vi "DataTXTFileInfo.vi"(9 "Language":u32, 11 "file path (dialog if empty)":path caption="文件路径 （空时为对话框）") -> (0 "路径输出":path, 1 "FileInfo":string, 2 "文件类型":string)   [LabVIEW 2015]
uses:
  <vilib>/regexp/Match Regular Expression.xnode
panel:
  out "匹配子字符串":string
  out "输出 2":string
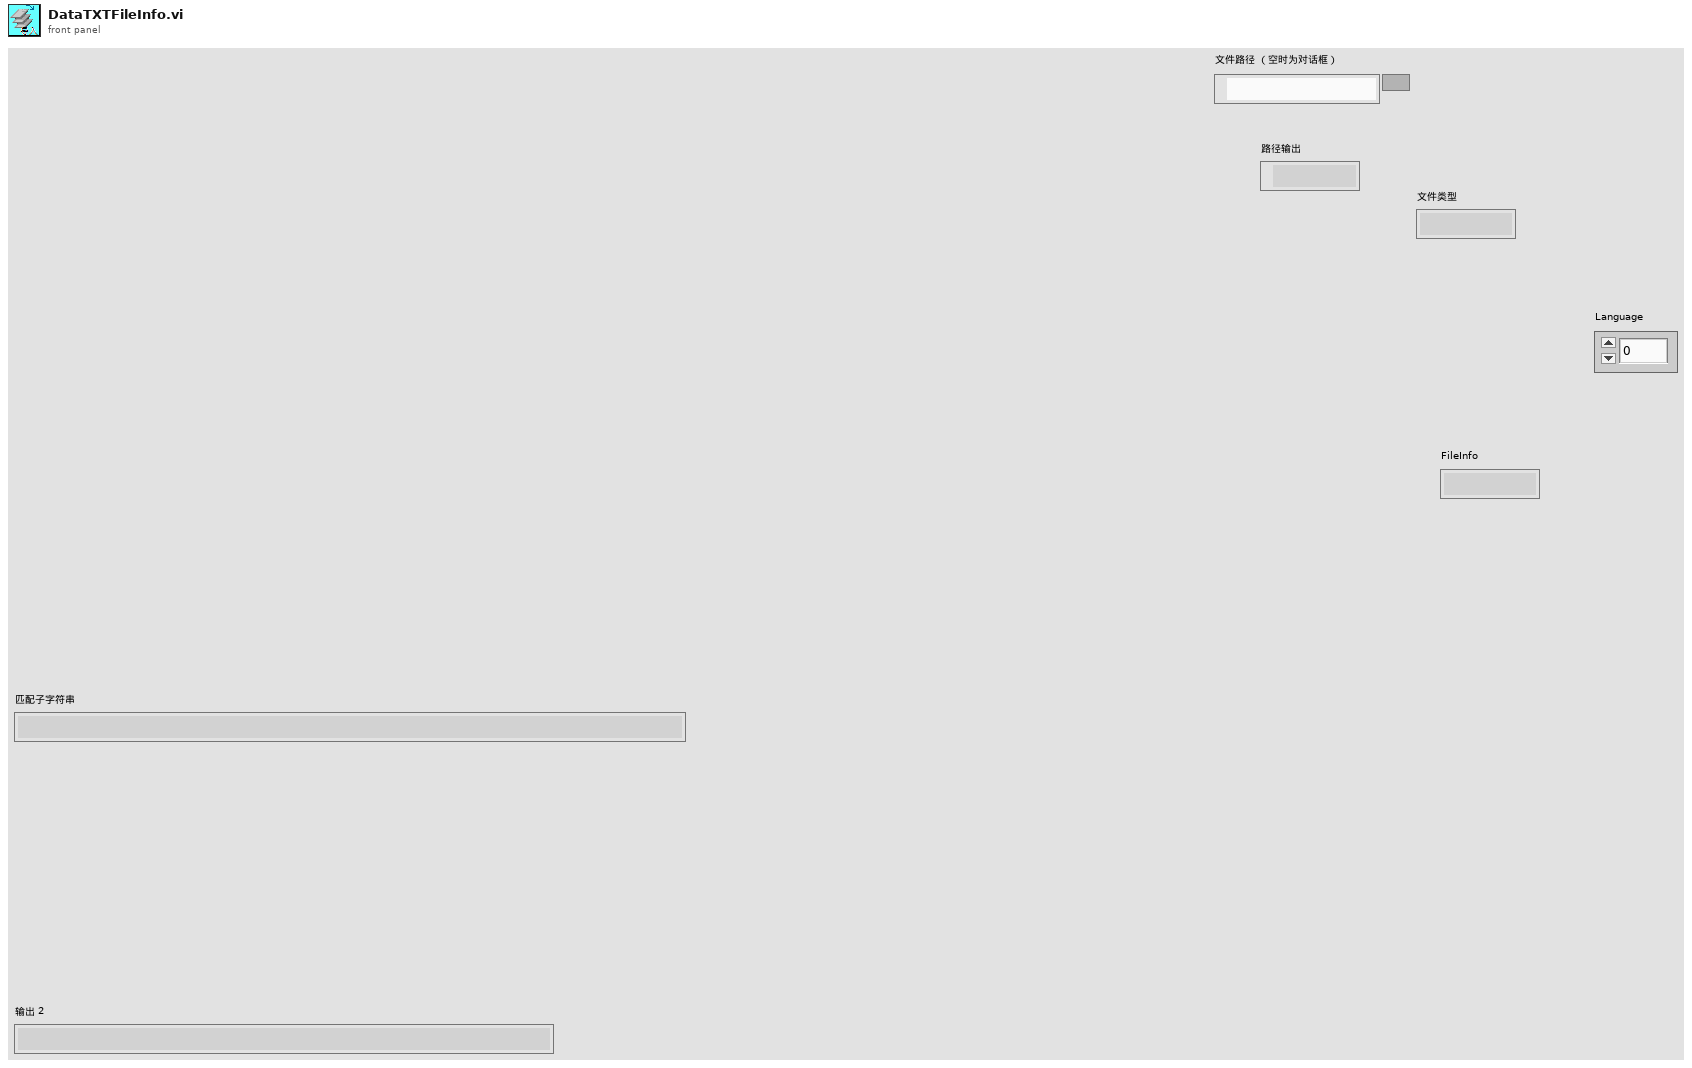
[diagram p1: front panel]
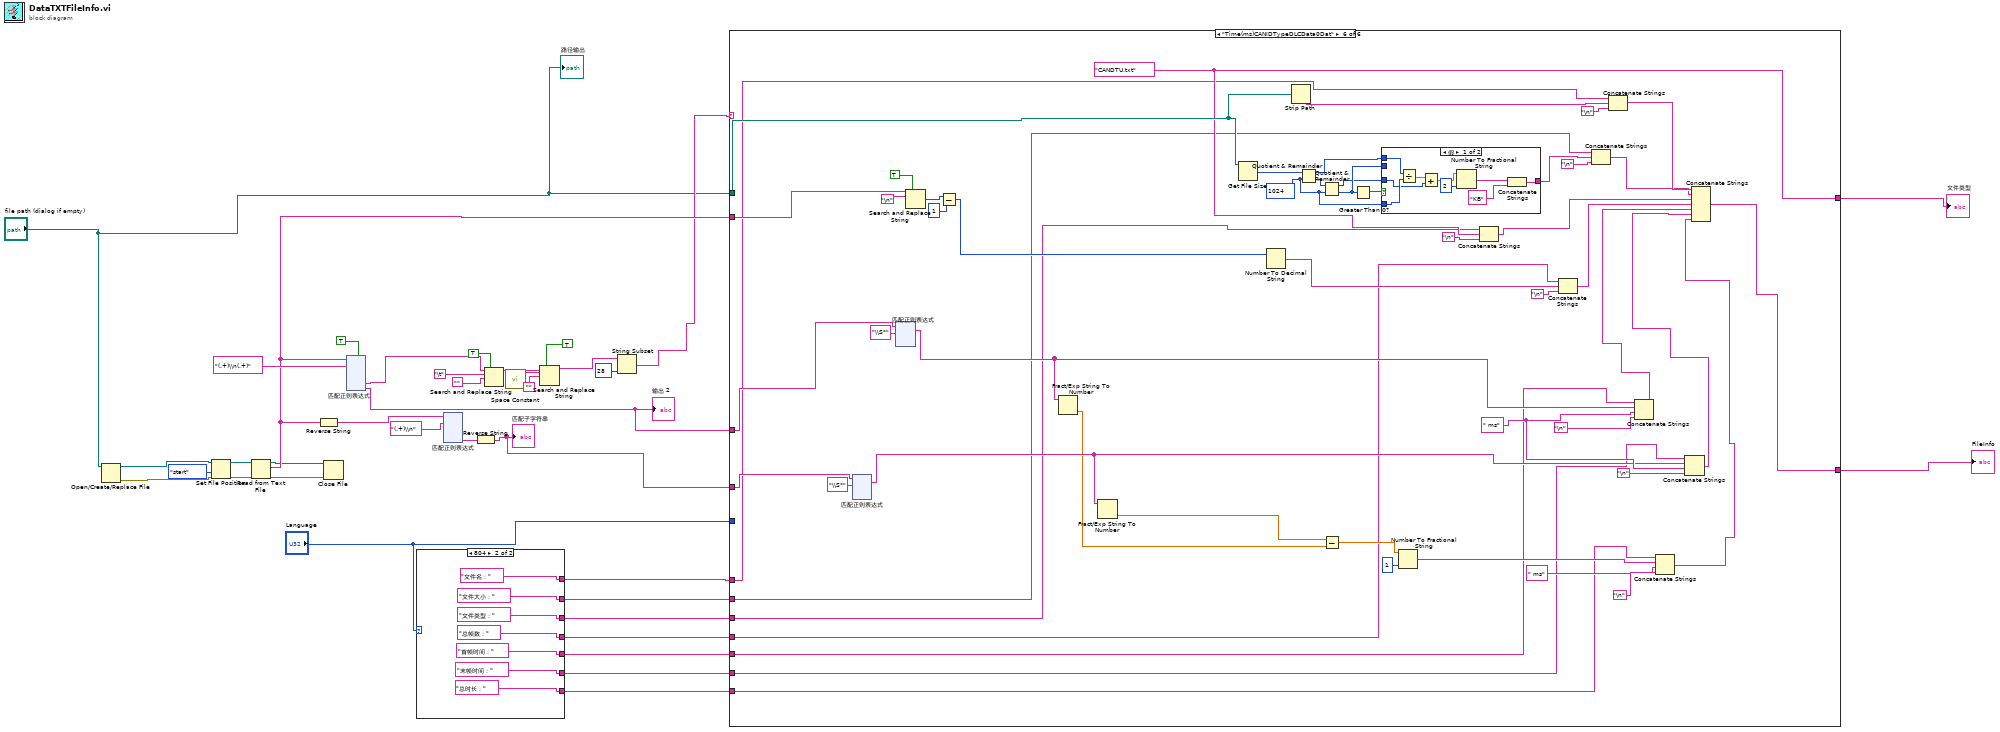
[diagram p0: block diagram]
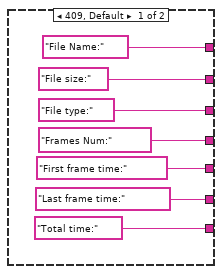
[diagram p2: hidden frame]
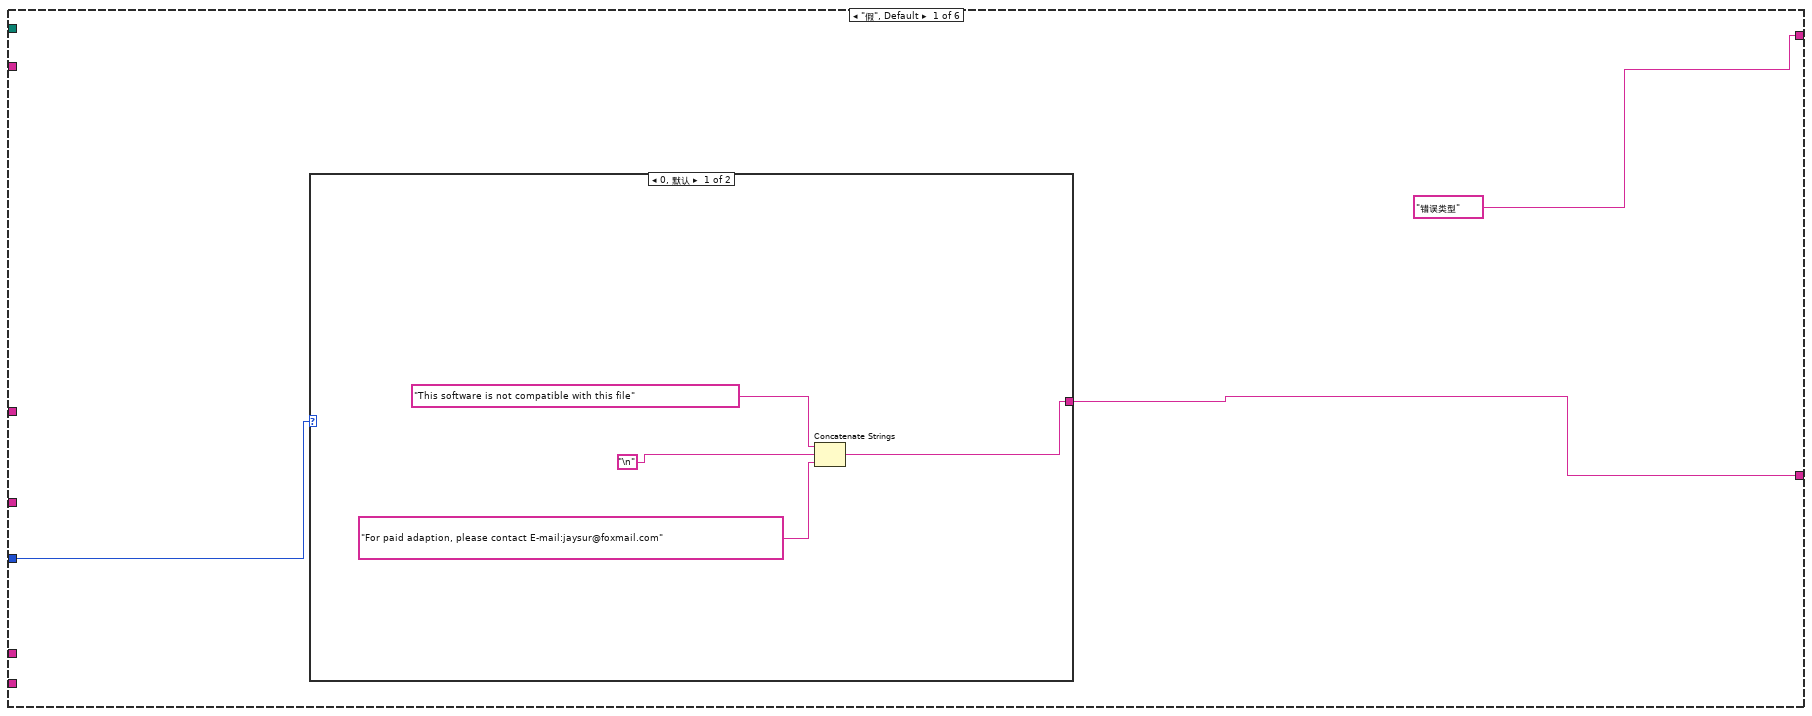
[diagram p3: hidden frame]
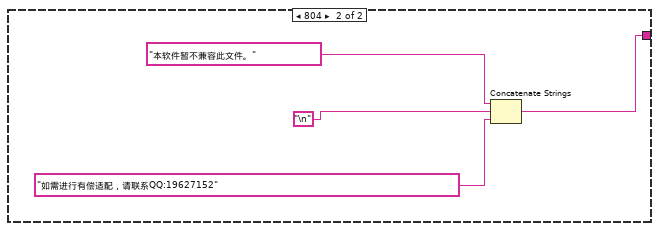
[diagram p4: hidden frame]
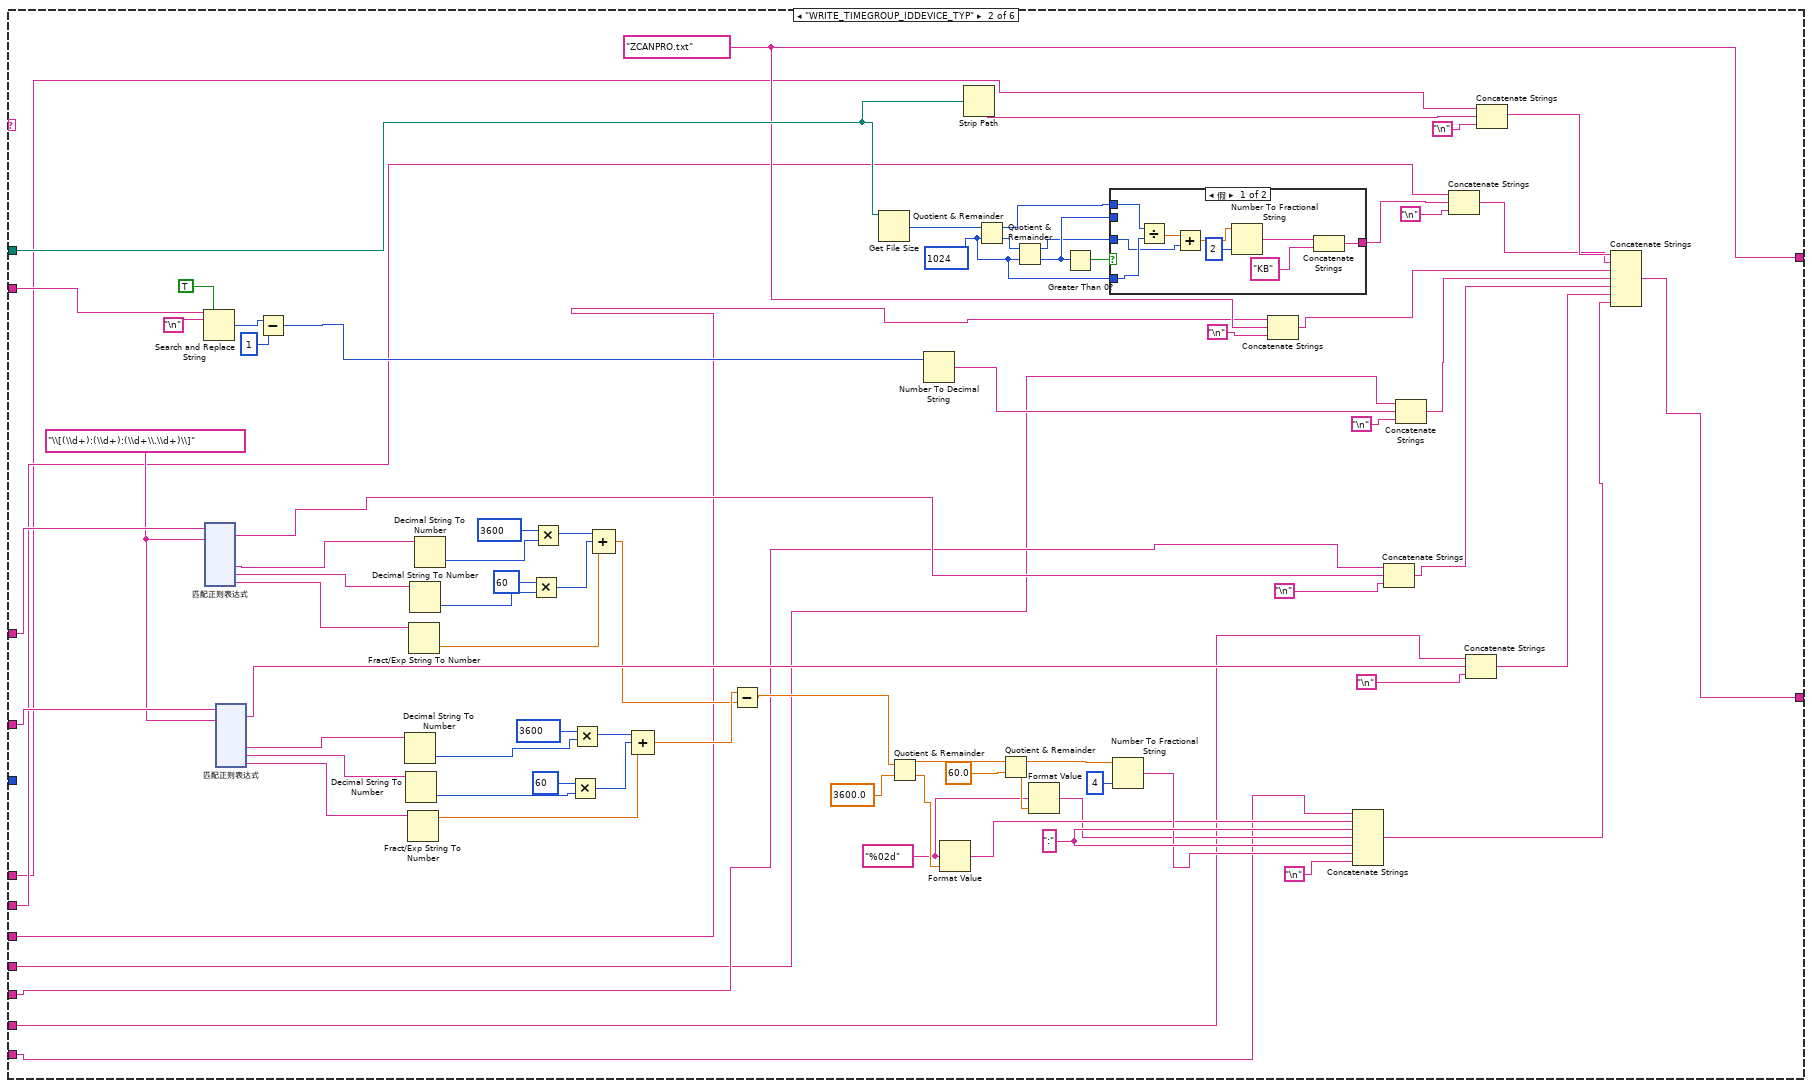
[diagram p5: hidden frame]
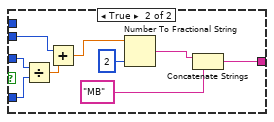
[diagram p6: hidden frame]
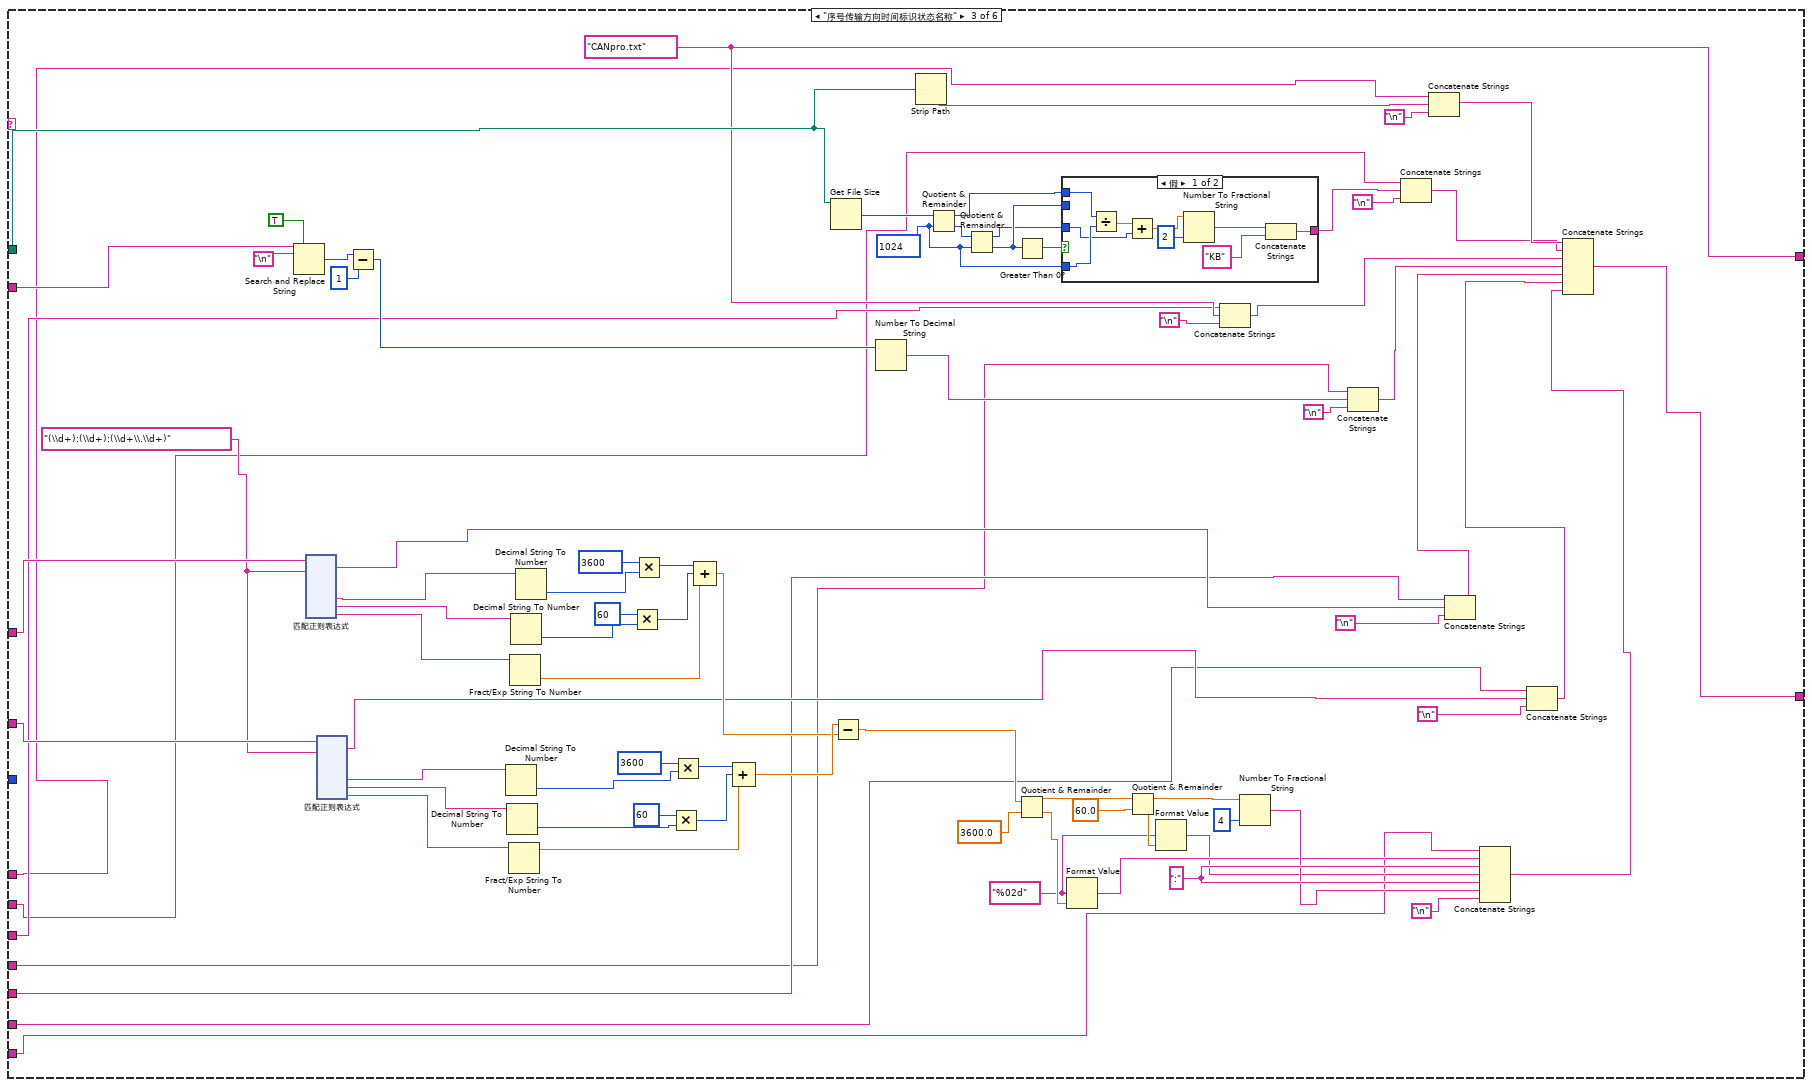
[diagram p7: hidden frame]
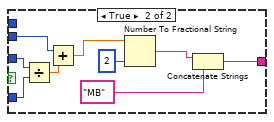
[diagram p8: hidden frame]
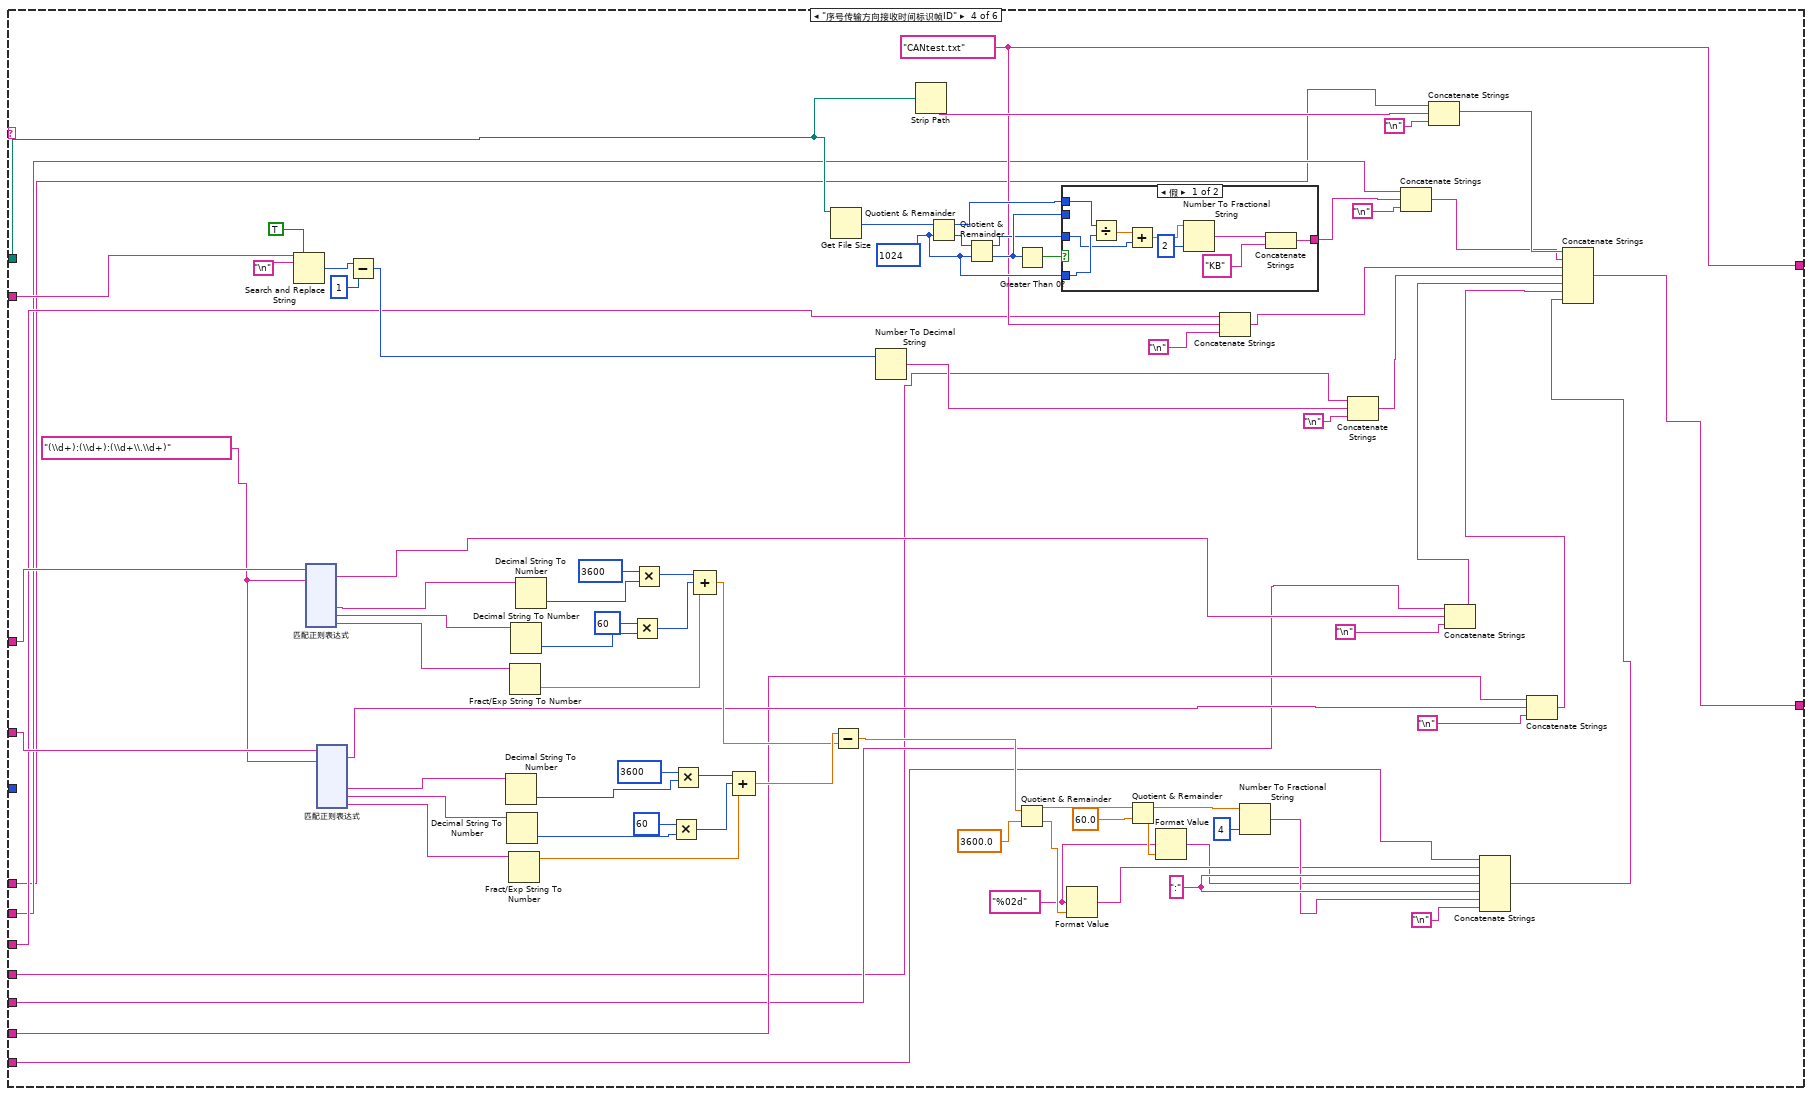
[diagram p9: hidden frame]
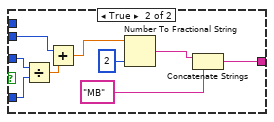
[diagram p10: hidden frame]
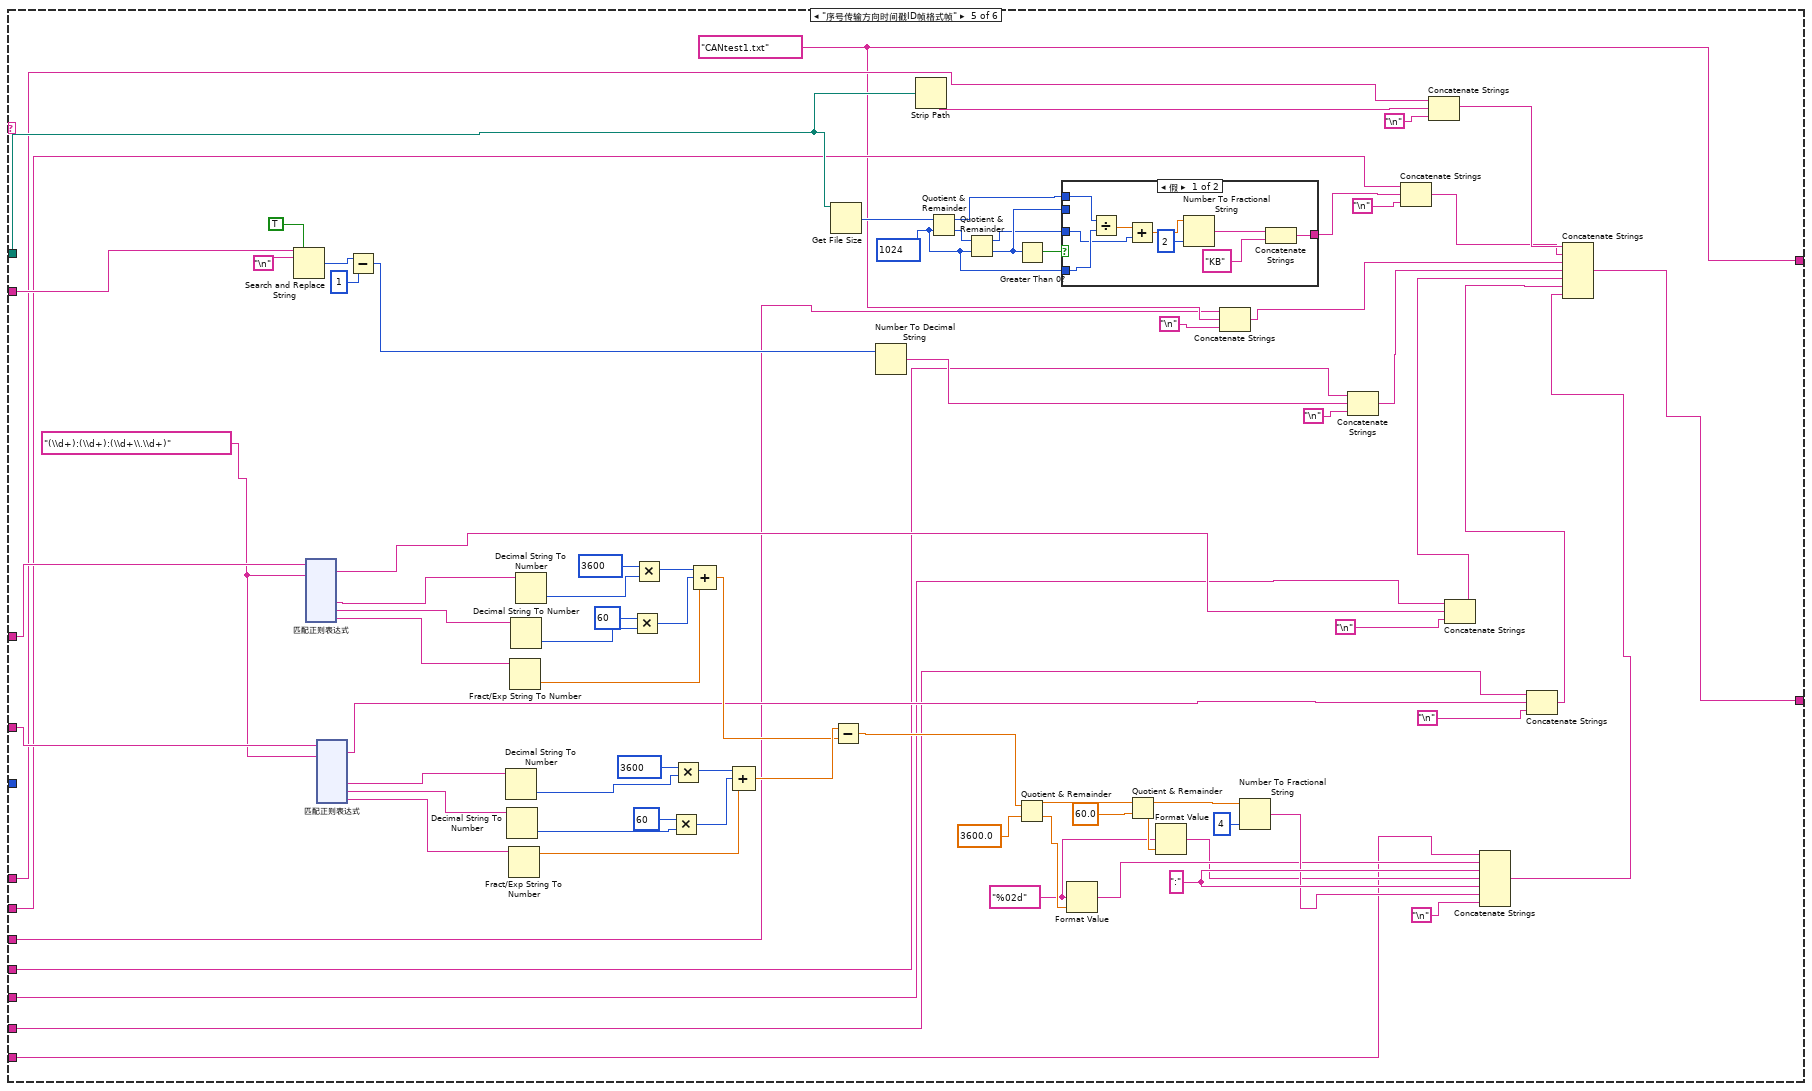
[diagram p11: hidden frame]
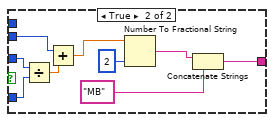
[diagram p12: hidden frame]
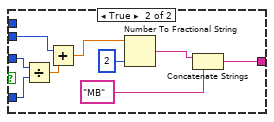
[diagram p13: hidden frame]
diagram:
  n1 = Open/Create/Replace File(file path (use dialog)="file path (dialog if empty)") -> (refnum out=w14:refnum<file>, error out=w13:errorcluster)  [unwired: 5 in, 1 out]
  n2 = Set File Position(refnum=w14, from (0:start)=enum16{"start", "end", "current"}."start" ("自（0:起始）"), error in=w13) -> (refnum out=w35:refnum<file>, error out=w33:errorcluster)  [unwired: 1 in]
  n3 = Read from Text File(file (use dialog)=w35, error in=w33) -> (refnum out=w11:refnum<file>, text=w17:string, error out=w12:errorcluster)  [unwired: 2 in, 1 out]
  n4 = Reverse String(1:w17) -> (0:w21:string)
  n5 = Close File(refnum=w11, error in=w12) -> ()  [unwired: 2 out]
  n6 = xnode "匹配正则表达式"("输入字符串"=w17, "正则表达式"="(.+)\\n(.+)", "多行？(F)"=TRUE) -> ("子匹配 1"=w28:string, "子匹配 2"=w15:string)  [unwired: 3 in, 5 out]
  "输出 2" <- w15
  n7 = case shown="804" "Language" {
    tunnel: ["Total time:" "总时长："] -> w7
    tunnel: ["Last frame time:" "末帧时间："] -> w6
    tunnel: ["First frame time:" "首帧时间："] -> w5
    tunnel: ["Frames Num:" "总帧数："] -> w4
    tunnel: ["File type:" "文件类型："] -> w3
    tunnel: ["File size:" "文件大小："] -> w2
    tunnel: ["File Name:" "文件名："] -> w1
    frame 409, Default {
    }
    frame 804 {
    }
  }
  n8 = xnode "匹配正则表达式"("输入字符串"=w21, "正则表达式"="(.+)\\n") -> ("子匹配 1"=w20:string)  [unwired: 4 in, 5 out]
  n9 = Reverse String(1:w20) -> (0:w9:string)
  "匹配子字符串" <- w9
  n10 = Search and Replace String(replace all?=TRUE ("替换全部？(F)"), input string=w28, search string="\t", replace string="") -> (result string=w26:string)  [unwired: 4 in, 3 out]
  n11 = call <vilib>:"Space Constant.vi"() -> ("String"=w25:string)
  n12 = Search and Replace String(replace all?=TRUE ("替换全部？(F)"), input string=w26, search string=w25, replace string="") -> (result string=w19:string)  [unwired: 4 in, 3 out]
  n13 = String Subset(string=w19, length (rest)=28 ("长度（剩余）")) -> (substring=w16:string)  [unwired: 1 in]
  n14 = case shown="\"Time(ms)CANIDTypeDLCData0Dat\"" w16 {
    tunnel: [w53 w109 w439 w773 w1107 w1432] -> w37
    tunnel: ["错误类型" w66 w404 w738 w1070 w1406] -> w36
    tunnel: "file path (dialog if empty)" -> [_ w105 w443 w777 w1111 w1433]
    tunnel: w17 -> [_ w100 w434 w768 w1102 w1427]
    tunnel: w15 -> [_ w96 w410 w744 w1078 w1407]
    tunnel: w9 -> [_ w98 w409 w743 w1077 w1408]
    tunnel: "Language" -> [w52 _ _ _ _ _]
    tunnel: w7 -> [_ w70 w400 w734 w1066 w1399]
    tunnel: w6 -> [_ w69 w399 w733 w1065 w1400]
    tunnel: w5 -> [_ w68 w398 w732 w1067 w1401]
    tunnel: w4 -> [_ w67 w397 w731 w1068 w1402]
    tunnel: w3 -> [_ w65 w403 w737 w1069 w1405]
    tunnel: w2 -> [_ w64 w402 w736 w1071 w1404]
    tunnel: w1 -> [_ w63 w401 w735 w1072 w1403]
    frame "假", Default {
      n15 = case shown="0, 默认" w52 {
        tunnel: [w55 w59] -> w53
        frame 0, Default {
          n16 = Concatenate Strings("This software is not compatible with this file", "\n", "For paid adaption, please contact E-mail:jaysur@foxmail.com") -> (w55:string)
        }
        frame 804 {
          n17 = Concatenate Strings("本软件暂不兼容此文件。", "\n", "如需进行有偿适配，请联系QQ:19627152") -> (w59:string)
        }
      }
    }
    frame "WRITE_TIMEGROUP_IDDEVICE_TYP" {
      w95 = "\\[(\\d+):(\\d+):(\\d+\\.\\d+)\\]"
      w114 = i64 1024 ("y")
      w131 = "%02d" ("格式字符串")
      w137 = ":"
      w66 = "ZCANPRO.txt"
      n18 = Search and Replace String(replace all?=TRUE ("替换全部？(F)"), input string=w100, search string="\n") -> (number of replacements=w102:i32)  [unwired: 5 in, 3 out]
      n19 = xnode "匹配正则表达式"("输入字符串"=w96, "正则表达式"=w95) -> ("所有匹配"=w94:string, "子匹配 1"=w93:string, "子匹配 2"=w92:string, "子匹配 3"=w91:string)  [unwired: 4 in, 4 out]
      n20 = xnode "匹配正则表达式"("输入字符串"=w98, "正则表达式"=w95) -> ("所有匹配"=w97:string, "子匹配 1"=w90:string, "子匹配 2"=w89:string, "子匹配 3"=w88:string)  [unwired: 4 in, 4 out]
      n21 = Subtract(x=w102, y=1) -> (x-y=w99:i32)
      n22 = Decimal String To Number(string=w90) -> (number=w76:i32)  [unwired: 2 in, 1 out]
      n23 = Decimal String To Number(string=w89) -> (number=w75:i32)  [unwired: 2 in, 1 out]
      n24 = Fract/Exp String To Number(string=w88) -> (number=w74:dbl)  [unwired: 3 in, 1 out]
      n25 = Fract/Exp String To Number(string=w91) -> (number=w81:dbl)  [unwired: 3 in, 1 out]
      n26 = Decimal String To Number(string=w92) -> (number=w87:i32)  [unwired: 2 in, 1 out]
      n27 = Decimal String To Number(string=w93) -> (number=w85:i32)  [unwired: 2 in, 1 out]
      n28 = Multiply(x=60, y=w87) -> (x*y=w82:i32)
      n29 = Multiply(x=3600, y=w85) -> (x*y=w83:i32)
      n30 = Multiply(x=60, y=w75) -> (x*y=w77:i32)
      n31 = Multiply(x=3600, y=w76) -> (x*y=w78:i32)
      n32 = Compound Arithmetic op=ADD(w83, w82, w81) -> (w72:dbl)
      n33 = Compound Arithmetic op=ADD(w78, w77, w74) -> (w73:dbl)
      n34 = Subtract(x=w73, y=w72) -> (x-y=w71:dbl)
      n35 = Get File Size(file=w105) -> (size (in bytes)=w117:i64)  [unwired: 1 in, 2 out]
      n36 = Quotient & Remainder(x=w71, y=3600.0) -> (x-y*floor(x/y)=w141:dbl, floor(x/y)=w134:dbl)
      n37 = Number To Decimal String(number=w99) -> (decimal integer string=w120:string)  [unwired: 1 in]
      n38 = Format Value(format string=w131, value (0)=w134) -> (output string=w135:string)  [unwired: 1 in]
      n39 = Strip Path(path=w105) -> (name=w127:string)  [unwired: 1 out]
      n40 = Quotient & Remainder(x=w117, y=w114) -> (x-y*floor(x/y)=w110:i64, floor(x/y)=w116:i64)
      n41 = Quotient & Remainder(x=w141, y=60.0) -> (x-y*floor(x/y)=w139:dbl, floor(x/y)=w133:dbl)
      n42 = Quotient & Remainder(x=w116, y=w114) -> (x-y*floor(x/y)=w112:i64, floor(x/y)=w113:i64)
      n43 = Format Value(format string=w131, value (0)=w133) -> (output string=w132:string)  [unwired: 1 in]
      n44 = Greater Than 0?(x=w113) -> (x > 0?=w115:bool)
      n45 = case shown="假" w115 {
        tunnel: w114 -> [w384 w394]
        tunnel: w113 -> [_ w392]
        tunnel: w112 -> [w382 w395]
        tunnel: [w387 w390] -> w111
        tunnel: w110 -> [w385 _]
        frame False {
          n46 = Divide(x=w385, y=w384) -> (x/y=w383:dbl)
          n47 = Add(x=w383, y=w382) -> (x+y=w381:dbl)
          n48 = Number To Fractional String(number=w381, precision (6)=i16 2 ("精度(6)")) -> (F-format string=w379:string)  [unwired: 2 in]
          n49 = Concatenate Strings(w379, "KB" ("字符串")) -> (w387:string)
        }
        frame True {
          n50 = Divide(x=w395, y=w394) -> (x/y=w393:dbl)
          n51 = Add(x=w392, y=w393) -> (x+y=w391:dbl)
          n52 = Number To Fractional String(number=w391, precision (6)=i16 2 ("精度(6)")) -> (F-format string=w389:string)  [unwired: 2 in]
          n53 = Concatenate Strings(w389, "MB") -> (w390:string)
        }
      }
      n54 = Number To Fractional String(number=w139, precision (6)=i16 4 ("精度(6)")) -> (F-format string=w136:string)  [unwired: 2 in]
      n55 = Concatenate Strings(w65, w66, "\n") -> (w124:string)
      n56 = Concatenate Strings(w70, w135, w137, w132, w137, w136, "\n") -> (w108:string)
      n57 = Concatenate Strings(w68, w94, "\n") -> (w106:string)
      n58 = Concatenate Strings(w67, w120, "\n") -> (w121:string)
      n59 = Concatenate Strings(w64, w111, "\n") -> (w118:string)
      n60 = Concatenate Strings(w69, w97, "\n") -> (w107:string)
      n61 = Concatenate Strings(w63, w127, "\n") -> (w126:string)
      n62 = Concatenate Strings(w126, w118, w124, w121, w106, w107, w108) -> (w109:string)
    }
    frame "序号传输方向时间标识状态名称" {
      w406 = "(\\d+):(\\d+):(\\d+\\.\\d+)"
      w448 = i64 1024 ("y")
      w465 = "%02d" ("格式字符串")
      w471 = ":"
      w404 = "CANpro.txt"
      n63 = Search and Replace String(replace all?=TRUE ("替换全部？(F)"), input string=w434, search string="\n") -> (number of replacements=w436:i32)  [unwired: 5 in, 3 out]
      n64 = xnode "匹配正则表达式"("输入字符串"=w410, "正则表达式"=w406) -> ("所有匹配"=w408:string, "子匹配 1"=w432:string, "子匹配 2"=w431:string, "子匹配 3"=w430:string)  [unwired: 4 in, 4 out]
      n65 = xnode "匹配正则表达式"("输入字符串"=w409, "正则表达式"=w406) -> ("所有匹配"=w407:string, "子匹配 1"=w429:string, "子匹配 2"=w428:string, "子匹配 3"=w427:string)  [unwired: 4 in, 4 out]
      n66 = Subtract(x=w436, y=1) -> (x-y=w433:i32)
      n67 = Decimal String To Number(string=w429) -> (number=w415:i32)  [unwired: 2 in, 1 out]
      n68 = Decimal String To Number(string=w428) -> (number=w414:i32)  [unwired: 2 in, 1 out]
      n69 = Fract/Exp String To Number(string=w427) -> (number=w413:dbl)  [unwired: 3 in, 1 out]
      n70 = Fract/Exp String To Number(string=w430) -> (number=w420:dbl)  [unwired: 3 in, 1 out]
      n71 = Decimal String To Number(string=w431) -> (number=w426:i32)  [unwired: 2 in, 1 out]
      n72 = Decimal String To Number(string=w432) -> (number=w424:i32)  [unwired: 2 in, 1 out]
      n73 = Multiply(x=60, y=w426) -> (x*y=w421:i32)
      n74 = Multiply(x=3600, y=w424) -> (x*y=w422:i32)
      n75 = Multiply(x=60, y=w414) -> (x*y=w416:i32)
      n76 = Multiply(x=3600, y=w415) -> (x*y=w417:i32)
      n77 = Compound Arithmetic op=ADD(w422, w421, w420) -> (w411:dbl)
      n78 = Compound Arithmetic op=ADD(w417, w416, w413) -> (w412:dbl)
      n79 = Get File Size(file=w443) -> (size (in bytes)=w451:i64)  [unwired: 1 in, 2 out]
      n80 = Subtract(x=w412, y=w411) -> (x-y=w405:dbl)
      n81 = Number To Decimal String(number=w433) -> (decimal integer string=w454:string)  [unwired: 1 in]
      n82 = Strip Path(path=w443) -> (name=w461:string)  [unwired: 1 out]
      n83 = Quotient & Remainder(x=w451, y=w448) -> (x-y*floor(x/y)=w444:i64, floor(x/y)=w450:i64)
      n84 = Quotient & Remainder(x=w450, y=w448) -> (x-y*floor(x/y)=w446:i64, floor(x/y)=w447:i64)
      n85 = Greater Than 0?(x=w447) -> (x > 0?=w449:bool)
      n86 = Quotient & Remainder(x=w405, y=3600.0) -> (x-y*floor(x/y)=w475:dbl, floor(x/y)=w468:dbl)
      n87 = case shown="假" w449 {
        tunnel: w448 -> [w718 w728]
        tunnel: w447 -> [_ w726]
        tunnel: w446 -> [w716 w729]
        tunnel: [w721 w724] -> w445
        tunnel: w444 -> [w719 _]
        frame False {
          n88 = Divide(x=w719, y=w718) -> (x/y=w717:dbl)
          n89 = Add(x=w717, y=w716) -> (x+y=w715:dbl)
          n90 = Number To Fractional String(number=w715, precision (6)=i16 2 ("精度(6)")) -> (F-format string=w713:string)  [unwired: 2 in]
          n91 = Concatenate Strings(w713, "KB" ("字符串")) -> (w721:string)
        }
        frame True {
          n92 = Divide(x=w729, y=w728) -> (x/y=w727:dbl)
          n93 = Add(x=w726, y=w727) -> (x+y=w725:dbl)
          n94 = Number To Fractional String(number=w725, precision (6)=i16 2 ("精度(6)")) -> (F-format string=w723:string)  [unwired: 2 in]
          n95 = Concatenate Strings(w723, "MB") -> (w724:string)
        }
      }
      n96 = Format Value(format string=w465, value (0)=w468) -> (output string=w469:string)  [unwired: 1 in]
      n97 = Quotient & Remainder(x=w475, y=60.0) -> (x-y*floor(x/y)=w473:dbl, floor(x/y)=w467:dbl)
      n98 = Format Value(format string=w465, value (0)=w467) -> (output string=w466:string)  [unwired: 1 in]
      n99 = Concatenate Strings(w403, w404, "\n") -> (w458:string)
      n100 = Number To Fractional String(number=w473, precision (6)=i16 4 ("精度(6)")) -> (F-format string=w470:string)  [unwired: 2 in]
      n101 = Concatenate Strings(w397, w454, "\n") -> (w455:string)
      n102 = Concatenate Strings(w402, w445, "\n") -> (w452:string)
      n103 = Concatenate Strings(w401, w461, "\n") -> (w460:string)
      n104 = Concatenate Strings(w398, w408, "\n") -> (w442:string)
      n105 = Concatenate Strings(w400, w469, w471, w466, w471, w470, "\n") -> (w440:string)
      n106 = Concatenate Strings(w399, w407, "\n") -> (w441:string)
      n107 = Concatenate Strings(w460, w452, w458, w455, w442, w441, w440) -> (w439:string)
    }
    frame "序号传输方向接收时间标识帧ID" {
      w740 = "(\\d+):(\\d+):(\\d+\\.\\d+)"
      w782 = i64 1024 ("y")
      w799 = "%02d" ("格式字符串")
      w805 = ":"
      w738 = "CANtest.txt"
      n108 = Search and Replace String(replace all?=TRUE ("替换全部？(F)"), input string=w768, search string="\n") -> (number of replacements=w770:i32)  [unwired: 5 in, 3 out]
      n109 = xnode "匹配正则表达式"("输入字符串"=w744, "正则表达式"=w740) -> ("所有匹配"=w742:string, "子匹配 1"=w766:string, "子匹配 2"=w765:string, "子匹配 3"=w764:string)  [unwired: 4 in, 4 out]
      n110 = xnode "匹配正则表达式"("输入字符串"=w743, "正则表达式"=w740) -> ("所有匹配"=w741:string, "子匹配 1"=w763:string, "子匹配 2"=w762:string, "子匹配 3"=w761:string)  [unwired: 4 in, 4 out]
      n111 = Subtract(x=w770, y=1) -> (x-y=w767:i32)
      n112 = Decimal String To Number(string=w763) -> (number=w749:i32)  [unwired: 2 in, 1 out]
      n113 = Decimal String To Number(string=w762) -> (number=w748:i32)  [unwired: 2 in, 1 out]
      n114 = Fract/Exp String To Number(string=w761) -> (number=w747:dbl)  [unwired: 3 in, 1 out]
      n115 = Fract/Exp String To Number(string=w764) -> (number=w754:dbl)  [unwired: 3 in, 1 out]
      n116 = Decimal String To Number(string=w765) -> (number=w760:i32)  [unwired: 2 in, 1 out]
      n117 = Decimal String To Number(string=w766) -> (number=w758:i32)  [unwired: 2 in, 1 out]
      n118 = Multiply(x=60, y=w760) -> (x*y=w755:i32)
      n119 = Multiply(x=3600, y=w758) -> (x*y=w756:i32)
      n120 = Multiply(x=60, y=w748) -> (x*y=w750:i32)
      n121 = Multiply(x=3600, y=w749) -> (x*y=w751:i32)
      n122 = Compound Arithmetic op=ADD(w756, w755, w754) -> (w745:dbl)
      n123 = Compound Arithmetic op=ADD(w751, w750, w747) -> (w746:dbl)
      n124 = Get File Size(file=w777) -> (size (in bytes)=w785:i64)  [unwired: 1 in, 2 out]
      n125 = Subtract(x=w746, y=w745) -> (x-y=w739:dbl)
      n126 = Number To Decimal String(number=w767) -> (decimal integer string=w788:string)  [unwired: 1 in]
      n127 = Strip Path(path=w777) -> (name=w795:string)  [unwired: 1 out]
      n128 = Quotient & Remainder(x=w785, y=w782) -> (x-y*floor(x/y)=w778:i64, floor(x/y)=w784:i64)
      n129 = Quotient & Remainder(x=w784, y=w782) -> (x-y*floor(x/y)=w780:i64, floor(x/y)=w781:i64)
      n130 = Greater Than 0?(x=w781) -> (x > 0?=w783:bool)
      n131 = Quotient & Remainder(x=w739, y=3600.0) -> (x-y*floor(x/y)=w809:dbl, floor(x/y)=w802:dbl)
      n132 = case shown="假" w783 {
        tunnel: w782 -> [w1052 w1062]
        tunnel: w781 -> [_ w1060]
        tunnel: w780 -> [w1050 w1063]
        tunnel: [w1055 w1058] -> w779
        tunnel: w778 -> [w1053 _]
        frame False {
          n133 = Divide(x=w1053, y=w1052) -> (x/y=w1051:dbl)
          n134 = Add(x=w1051, y=w1050) -> (x+y=w1049:dbl)
          n135 = Number To Fractional String(number=w1049, precision (6)=i16 2 ("精度(6)")) -> (F-format string=w1047:string)  [unwired: 2 in]
          n136 = Concatenate Strings(w1047, "KB" ("字符串")) -> (w1055:string)
        }
        frame True {
          n137 = Divide(x=w1063, y=w1062) -> (x/y=w1061:dbl)
          n138 = Add(x=w1060, y=w1061) -> (x+y=w1059:dbl)
          n139 = Number To Fractional String(number=w1059, precision (6)=i16 2 ("精度(6)")) -> (F-format string=w1057:string)  [unwired: 2 in]
          n140 = Concatenate Strings(w1057, "MB") -> (w1058:string)
        }
      }
      n141 = Format Value(format string=w799, value (0)=w802) -> (output string=w803:string)  [unwired: 1 in]
      n142 = Quotient & Remainder(x=w809, y=60.0) -> (x-y*floor(x/y)=w807:dbl, floor(x/y)=w801:dbl)
      n143 = Format Value(format string=w799, value (0)=w801) -> (output string=w800:string)  [unwired: 1 in]
      n144 = Concatenate Strings(w737, w738, "\n") -> (w792:string)
      n145 = Number To Fractional String(number=w807, precision (6)=i16 4 ("精度(6)")) -> (F-format string=w804:string)  [unwired: 2 in]
      n146 = Concatenate Strings(w731, w788, "\n") -> (w789:string)
      n147 = Concatenate Strings(w736, w779, "\n") -> (w786:string)
      n148 = Concatenate Strings(w735, w795, "\n") -> (w794:string)
      n149 = Concatenate Strings(w732, w742, "\n") -> (w776:string)
      n150 = Concatenate Strings(w734, w803, w805, w800, w805, w804, "\n") -> (w774:string)
      n151 = Concatenate Strings(w733, w741, "\n") -> (w775:string)
      n152 = Concatenate Strings(w794, w786, w792, w789, w776, w775, w774) -> (w773:string)
    }
    frame "序号传输方向时间戳ID帧格式帧" {
      w1074 = "(\\d+):(\\d+):(\\d+\\.\\d+)"
      w1116 = i64 1024 ("y")
      w1133 = "%02d" ("格式字符串")
      w1139 = ":"
      w1070 = "CANtest1.txt"
      n153 = Search and Replace String(replace all?=TRUE ("替换全部？(F)"), input string=w1102, search string="\n") -> (number of replacements=w1104:i32)  [unwired: 5 in, 3 out]
      n154 = xnode "匹配正则表达式"("输入字符串"=w1078, "正则表达式"=w1074) -> ("所有匹配"=w1076:string, "子匹配 1"=w1100:string, "子匹配 2"=w1099:string, "子匹配 3"=w1098:string)  [unwired: 4 in, 4 out]
      n155 = xnode "匹配正则表达式"("输入字符串"=w1077, "正则表达式"=w1074) -> ("所有匹配"=w1075:string, "子匹配 1"=w1097:string, "子匹配 2"=w1096:string, "子匹配 3"=w1095:string)  [unwired: 4 in, 4 out]
      n156 = Subtract(x=w1104, y=1) -> (x-y=w1101:i32)
      n157 = Decimal String To Number(string=w1097) -> (number=w1083:i32)  [unwired: 2 in, 1 out]
      n158 = Decimal String To Number(string=w1096) -> (number=w1082:i32)  [unwired: 2 in, 1 out]
      n159 = Fract/Exp String To Number(string=w1095) -> (number=w1081:dbl)  [unwired: 3 in, 1 out]
      n160 = Fract/Exp String To Number(string=w1098) -> (number=w1088:dbl)  [unwired: 3 in, 1 out]
      n161 = Decimal String To Number(string=w1099) -> (number=w1094:i32)  [unwired: 2 in, 1 out]
      n162 = Decimal String To Number(string=w1100) -> (number=w1092:i32)  [unwired: 2 in, 1 out]
      n163 = Multiply(x=60, y=w1094) -> (x*y=w1089:i32)
      n164 = Multiply(x=3600, y=w1092) -> (x*y=w1090:i32)
      n165 = Multiply(x=60, y=w1082) -> (x*y=w1084:i32)
      n166 = Multiply(x=3600, y=w1083) -> (x*y=w1085:i32)
      n167 = Compound Arithmetic op=ADD(w1090, w1089, w1088) -> (w1079:dbl)
      n168 = Compound Arithmetic op=ADD(w1085, w1084, w1081) -> (w1080:dbl)
      n169 = Get File Size(file=w1111) -> (size (in bytes)=w1119:i64)  [unwired: 1 in, 2 out]
      n170 = Subtract(x=w1080, y=w1079) -> (x-y=w1073:dbl)
      n171 = Number To Decimal String(number=w1101) -> (decimal integer string=w1122:string)  [unwired: 1 in]
      n172 = Strip Path(path=w1111) -> (name=w1129:string)  [unwired: 1 out]
      n173 = Quotient & Remainder(x=w1119, y=w1116) -> (x-y*floor(x/y)=w1112:i64, floor(x/y)=w1118:i64)
      n174 = Quotient & Remainder(x=w1118, y=w1116) -> (x-y*floor(x/y)=w1114:i64, floor(x/y)=w1115:i64)
      n175 = Greater Than 0?(x=w1115) -> (x > 0?=w1117:bool)
      n176 = Quotient & Remainder(x=w1073, y=3600.0) -> (x-y*floor(x/y)=w1143:dbl, floor(x/y)=w1136:dbl)
      n177 = case shown="假" w1117 {
        tunnel: w1116 -> [w1386 w1396]
        tunnel: w1115 -> [_ w1394]
        tunnel: w1114 -> [w1384 w1397]
        tunnel: [w1389 w1392] -> w1113
        tunnel: w1112 -> [w1387 _]
        frame False {
          n178 = Divide(x=w1387, y=w1386) -> (x/y=w1385:dbl)
          n179 = Add(x=w1385, y=w1384) -> (x+y=w1383:dbl)
          n180 = Number To Fractional String(number=w1383, precision (6)=i16 2 ("精度(6)")) -> (F-format string=w1381:string)  [unwired: 2 in]
          n181 = Concatenate Strings(w1381, "KB" ("字符串")) -> (w1389:string)
        }
        frame True {
          n182 = Divide(x=w1397, y=w1396) -> (x/y=w1395:dbl)
          n183 = Add(x=w1394, y=w1395) -> (x+y=w1393:dbl)
          n184 = Number To Fractional String(number=w1393, precision (6)=i16 2 ("精度(6)")) -> (F-format string=w1391:string)  [unwired: 2 in]
          n185 = Concatenate Strings(w1391, "MB") -> (w1392:string)
        }
      }
      n186 = Format Value(format string=w1133, value (0)=w1136) -> (output string=w1137:string)  [unwired: 1 in]
      n187 = Quotient & Remainder(x=w1143, y=60.0) -> (x-y*floor(x/y)=w1141:dbl, floor(x/y)=w1135:dbl)
      n188 = Format Value(format string=w1133, value (0)=w1135) -> (output string=w1134:string)  [unwired: 1 in]
      n189 = Concatenate Strings(w1069, w1070, "\n") -> (w1126:string)
      n190 = Number To Fractional String(number=w1141, precision (6)=i16 4 ("精度(6)")) -> (F-format string=w1138:string)  [unwired: 2 in]
      n191 = Concatenate Strings(w1068, w1122, "\n") -> (w1123:string)
      n192 = Concatenate Strings(w1071, w1113, "\n") -> (w1120:string)
      n193 = Concatenate Strings(w1072, w1129, "\n") -> (w1128:string)
      n194 = Concatenate Strings(w1067, w1076, "\n") -> (w1110:string)
      n195 = Concatenate Strings(w1066, w1137, w1139, w1134, w1139, w1138, "\n") -> (w1108:string)
      n196 = Concatenate Strings(w1065, w1075, "\n") -> (w1109:string)
      n197 = Concatenate Strings(w1128, w1120, w1126, w1123, w1110, w1109, w1108) -> (w1107:string)
    }
    frame "Time(ms)CANIDTypeDLCData0Dat" {
      w1420 = " ms"
      w1438 = i64 1024 ("y")
      w1406 = "CANDTU.txt"
      n198 = xnode "匹配正则表达式"("输入字符串"=w1408, "正则表达式"="\\S*") -> ("所有匹配"=w1418:string)  [unwired: 4 in, 4 out]
      n199 = xnode "匹配正则表达式"("输入字符串"=w1407, "正则表达式"="\\S*") -> ("所有匹配"=w1419:string)  [unwired: 4 in, 4 out]
      n200 = Search and Replace String(replace all?=TRUE ("替换全部？(F)"), input string=w1427, search string="\n") -> (number of replacements=w1429:i32)  [unwired: 5 in, 3 out]
      n201 = Subtract(x=w1429, y=1) -> (x-y=w1426:i32)
      n202 = Fract/Exp String To Number(string=w1419) -> (number=w1416:dbl)  [unwired: 3 in, 1 out]
      n203 = Fract/Exp String To Number(string=w1418) -> (number=w1417:dbl)  [unwired: 3 in, 1 out]
      n204 = Get File Size(file=w1433) -> (size (in bytes)=w1441:i64)  [unwired: 1 in, 2 out]
      n205 = Number To Decimal String(number=w1426) -> (decimal integer string=w1444:string)  [unwired: 1 in]
      n206 = Strip Path(path=w1433) -> (name=w1451:string)  [unwired: 1 out]
      n207 = Quotient & Remainder(x=w1441, y=w1438) -> (x-y*floor(x/y)=w1434:i64, floor(x/y)=w1440:i64)
      n208 = Quotient & Remainder(x=w1440, y=w1438) -> (x-y*floor(x/y)=w1436:i64, floor(x/y)=w1437:i64)
      n209 = Subtract(x=w1417, y=w1416) -> (x-y=w1415:dbl)
      n210 = Greater Than 0?(x=w1437) -> (x > 0?=w1439:bool)
      n211 = case shown="假" w1439 {
        tunnel: w1438 -> [w1685 w1695]
        tunnel: w1437 -> [_ w1693]
        tunnel: w1436 -> [w1683 w1696]
        tunnel: [w1688 w1691] -> w1435
        tunnel: w1434 -> [w1686 _]
        frame False {
          n212 = Divide(x=w1686, y=w1685) -> (x/y=w1684:dbl)
          n213 = Add(x=w1684, y=w1683) -> (x+y=w1682:dbl)
          n214 = Number To Fractional String(number=w1682, precision (6)=i16 2 ("精度(6)")) -> (F-format string=w1680:string)  [unwired: 2 in]
          n215 = Concatenate Strings(w1680, "KB" ("字符串")) -> (w1688:string)
        }
        frame True {
          n216 = Divide(x=w1696, y=w1695) -> (x/y=w1694:dbl)
          n217 = Add(x=w1693, y=w1694) -> (x+y=w1692:dbl)
          n218 = Number To Fractional String(number=w1692, precision (6)=i16 2 ("精度(6)")) -> (F-format string=w1690:string)  [unwired: 2 in]
          n219 = Concatenate Strings(w1690, "MB") -> (w1691:string)
        }
      }
      n220 = Number To Fractional String(number=w1415, precision (6)=i16 1 ("精度(6)")) -> (F-format string=w1413:string)  [unwired: 2 in]
      n221 = Concatenate Strings(w1405, w1406, "\n") -> (w1448:string)
      n222 = Concatenate Strings(w1402, w1444, "\n") -> (w1445:string)
      n223 = Concatenate Strings(w1404, w1435, "\n") -> (w1442:string)
      n224 = Concatenate Strings(w1403, w1451, "\n") -> (w1450:string)
      n225 = Concatenate Strings(w1401, w1419, w1420, "\n") -> (w1409:string)
      n226 = Concatenate Strings(w1399, w1413, " ms", "\n") -> (w1411:string)
      n227 = Concatenate Strings(w1400, w1418, w1420, "\n") -> (w1410:string)
      n228 = Concatenate Strings(w1450, w1442, w1448, w1445, w1409, w1410, w1411) -> (w1432:string)
    }
  }
  "FileInfo" <- w37
  "文件类型" <- w36
  "路径输出" <- "file path (dialog if empty)"
